vi "AMZ_S3_APIHLP_Correct leading slash in path and query string.vi"(4 "Path and query string in":string) -> (1 "Corrected Path and query string":string)   [LabVIEW 2015, in "LV Interface for Amazon S3.lvlib"]
uses:
  LV Interface for Amazon S3.lvlib
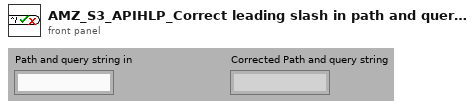
[diagram p1: front panel]
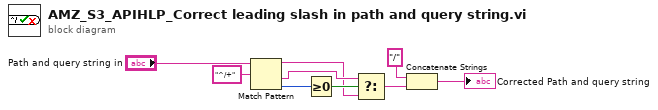
[diagram p0: block diagram]
diagram:
  n1 = Match Pattern(string="Path and query string in", regular expression="^/+") -> (before substring=w4:string, after substring=w5:string, offset past match=w7:i32)  [unwired: 1 in, 1 out]
  n2 = Greater Or Equal To 0?(x=w7) -> (x >= 0?=w6:bool)
  n3 = Select(t=w5, s=w6, f=w4) -> (s? t:f=w3:string)
  n4 = Concatenate Strings("/" ("string"), w3) -> (→"Corrected Path and query string":string)
